vi "read_temp.vi"() -> (0 "Temperature (C)":dbl)   [LabVIEW 2011]
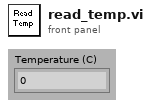
[diagram p1: front panel]
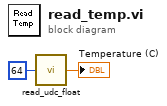
[diagram p0: block diagram]
diagram:
  n1 = call "read_udc_float.vi"("Hex Address"=u16 64) -> ("Value"=→"Temperature (C)":dbl)
